vi "GET Stop Event.vi"() -> (0 "Stop Event":refnum<user-event>)   [LabVIEW 2013]
uses:
  Functional Globals/Action.ctl
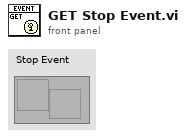
[diagram p1: front panel]
types:
  T1 = typedef "Action.ctl" = enum16{"GET", "PUT", "DELETE"}
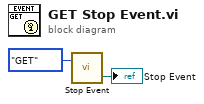
[diagram p0: block diagram]
diagram:
  n1 = call "Stop Event.vi"("Action"=Action."GET") -> ("Output"=→"Stop Event":refnum<user-event>)  [unwired: 2 in]
